vi "Open Camera.vi"(8 "error in":errorcluster, 10 "Camera":T1, 11 "Gantry in":refnum<class "Gantry Class.lvclass">) -> (0 "error out":errorcluster, 2 "Camera Out":T1, 3 "Gantry out":refnum<class "Gantry Class.lvclass">)   [LabVIEW 2011, in "Gantry Class.lvclass"]
uses:
  Gantry Class.lvclass
  Type Definitions/Gantry_Camera.ctl
  <vilib>/userdefined/High Color/IMAQdx.ctl
  Config Manager Class/Config Manager Class.lvclass
  <vilib>/vision/driver/NI_Vision_Acquisition_Software.lvlib
panel:
  # "This is a utility function to Open a camera for \"grab\"\nand, if necessary close an already open camera in the\nsame group.\n\nDo not use this function directly! Instead use the \"Get Image\"\nVI."
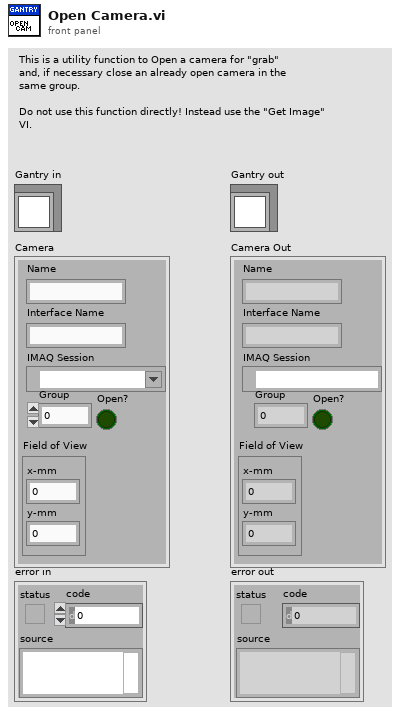
[diagram p1: front panel]
types:
  T1 = typedef "Gantry_Camera.ctl" = cluster{"Name":string, "IMAQ Session":T2, "Group":u32, "Open?":bool, "Interface Name":string, "Field of View":cluster{"x-mm":dbl, "y-mm":dbl}}
  T2 = typedef "IMAQdx.ctl" = refnum<k21>
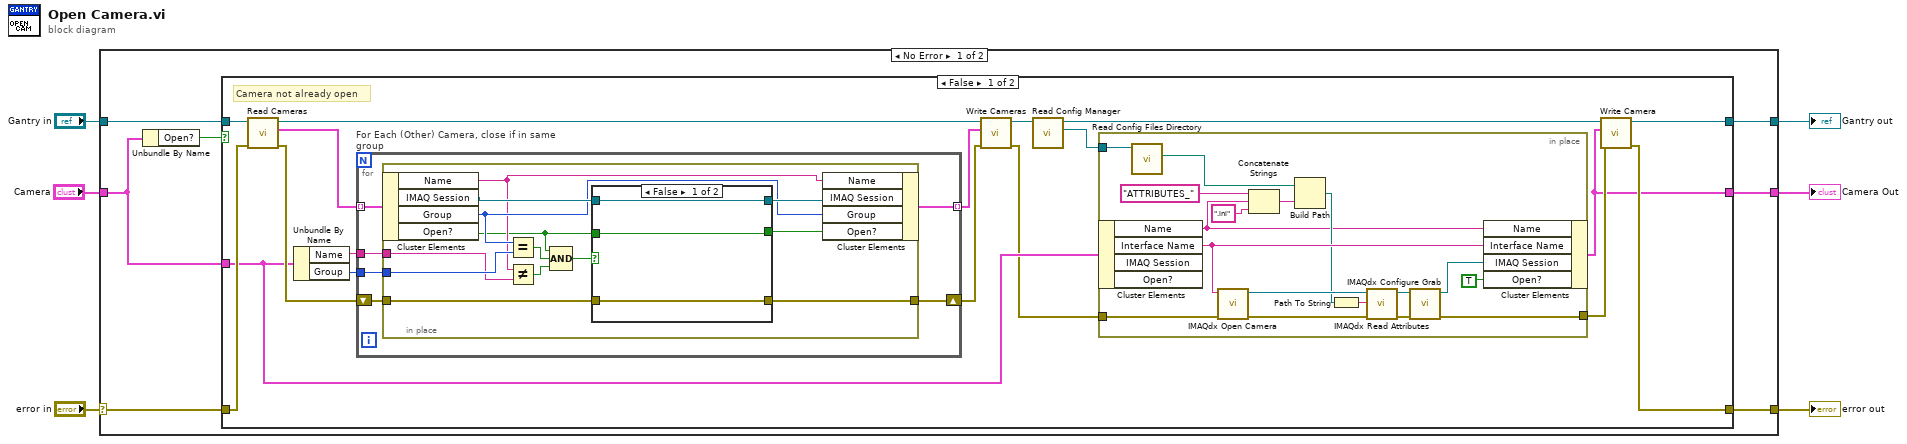
[diagram p0: block diagram]
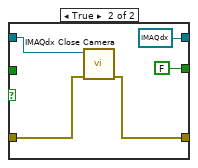
[diagram p2: hidden frame]
diagram:
  n1 = case shown="No Error" "error in" {
    selector: "error in" -> [w9 w81]
    tunnel: [w11 w81] -> w5
    tunnel: [w12 w80] -> w3
    tunnel: "Gantry in" -> [w10 w80]
    tunnel: "Camera" -> [w8 w79]
    tunnel: [w7 w79] -> w1
    frame No Error {
      n2 = Unbundle By Name(w8) -> ("Open?"=w13:bool)
      n3 = case shown="False" w13 {
        tunnel: w10 -> [w31 w78]
        tunnel: [w19 w78] -> w12
        tunnel: w8 -> [w22 w76]
        tunnel: w9 -> [w28 w77]
        tunnel: [w18 w77] -> w11
        tunnel: [w17 w76] -> w7
        frame False {
          # "Camera not already open"
          n4 = call-dynamic "Read Cameras.vi"("error in (no error)"=w28, "Gantry Class in"=w31) -> ("error out"=w26:errorcluster, "Cameras"=w30:T1[], "Gantry Class out"=w24:refnum<class "Gantry Class.lvclass">)  [unwired: 7 in]
          n5 = Unbundle By Name(w22) -> ("Name"=w27:string, "Group"=w29:u32)
          n6 = for "For Each (Other) Camera, close if in same group" {
            tunnel: w30 -> [w51] mode=indexing
            tunnel: w29 -> [w54]
            tunnel: w27 -> [w53]
            tunnel: [w50] -> w25 mode=indexing
            shift-right: [w49] -> w23
            shift-left: w26 -> [w52]
            n7 = in-place {
              in-place-border: w54 -> [w67]
              in-place-border: w53 -> [w66]
              in-place-border: w52 -> [w62]
              in-place-border: [w55] -> w49
              n8 = in-place-cluster #1(w51) -> ("Name"=w57:string, "IMAQ Session"=w61:T2, "Group"=w58:u32, "Open?"=w56:bool)
              n9 = Equal?(x=w58, y=w67) -> (x = y?=w64:bool)
              n10 = Not Equal?(x=w57, y=w66) -> (x != y?=w65:bool)
              n11 = Compound Arithmetic op=AND(w56, w64, w65) -> (w63:bool)
              n12 = case shown="False" w63 {
                tunnel: w61 -> [w69 w75]
                tunnel: w62 -> [w70 w74]
                tunnel: [w70 w73] -> w55
                tunnel: [w69 T2 refnum ("IMAQ Session")] -> w60
                tunnel: [w68 FALSE ("Open?")] -> w59
                tunnel: w56 -> [w68 _]
                frame False {
                }
                frame True {
                  n13 = call <vilib>:"IMAQdx Close Camera.vi"("error in"=w74, "Session In"=w75) -> ("error out"=w73:errorcluster)  [unwired: 9 in]
                }
              }
              n14 = in-place-cluster #1("Name"=w57, "IMAQ Session"=w60, "Group"=w58, "Open?"=w59) -> (w50:T1)
            }
          }
          n15 = call-dynamic "Write Cameras.vi"("error in (no error)"=w23, "Cameras"=w25, "Gantry Class in"=w24) -> ("error out"=w21:errorcluster, "Gantry Class out"=w16:refnum<class "Gantry Class.lvclass">)  [unwired: 7 in]
          n16 = call-dynamic "Read Config Manager.vi"("Gantry in"=w16) -> ("Config Manager"=w14:refnum<class "Config Manager Class.lvclass">, "Gantry out"=w15:refnum<class "Gantry Class.lvclass">)  [unwired: 8 in, 1 out]
          n17 = in-place "Open New Camera" {
            in-place-border: w21 -> [w48]
            in-place-border: [w44] -> w20
            in-place-border: w14 -> [w33]
            n18 = in-place-cluster #2(w22) -> ("Name"=w34:string, "Interface Name"=w45:string)  [unwired: 2 out]
            n19 = call-dynamic "Read Config Files Directory.vi"("Config Manager Class in"=w33) -> ("Config Files Directory"=w32:path)  [unwired: 8 in, 2 out]
            n20 = call <vilib>:"IMAQdx Open Camera.vi"("error in"=w48, "Session In"=w45) -> ("error out"=w38:errorcluster, "Session Out"=w37:T2)  [unwired: 8 in]
            n21 = Concatenate Strings("ATTRIBUTES_" ("string"), w34, ".ini" ("string")) -> (w42:string)
            n22 = Build Path(base path=w32, name or relative path=w42) -> (appended path=w35:path)
            n23 = Path To String(path=w35) -> (string=w36:string)
            n24 = call <vilib>:"IMAQdx Read Attributes.vi"("error in"=w38, "Filename"=w36, "Session In"=w37) -> ("error out"=w39:errorcluster, "Session Out"=w40:T2)  [unwired: 7 in]
            n25 = call <vilib>:"IMAQdx Configure Grab.vi"("error in"=w39, "Session In"=w40) -> ("error out"=w44:errorcluster, "Session Out"=w46:T2)  [unwired: 8 in]
            n26 = in-place-cluster #2("Name"=w34, "Interface Name"=w45, "IMAQ Session"=w46, "Open?"=TRUE) -> (w17:T1)
          }
          n27 = call-dynamic "Write Camera.vi"("error in (no error)"=w20, "Camera"=w17, "Gantry Class in"=w15) -> ("error out"=w18:errorcluster, "Gantry Class out"=w19:refnum<class "Gantry Class.lvclass">)  [unwired: 6 in]
        }
        frame True {
          # "Camera already open, do nothing"
        }
      }
    }
    frame Error {
    }
  }
  "error out" <- w5
  "Gantry out" <- w3
  "Camera Out" <- w1
